vi "Load Preset.vi"(8 "error in (no error)":errorcluster, 10 "Preset Name":string, 11 "Config":T3) -> (0 "error out":errorcluster, 1 "Dump Stat":T1, 2 "Levels Available":i32, 3 "Levels":T2, 5 "No Oxy?":bool)   [LabVIEW 2021]
uses:
  <vilib>/Utility/config.llb/Config Data RefNum.ctl
  CTLs/Dump Stat.ctl
  <vilib>/Utility/config.llb/Read Key (I32).vi
  <vilib>/Utility/config.llb/NI_LVConfig.lvlib
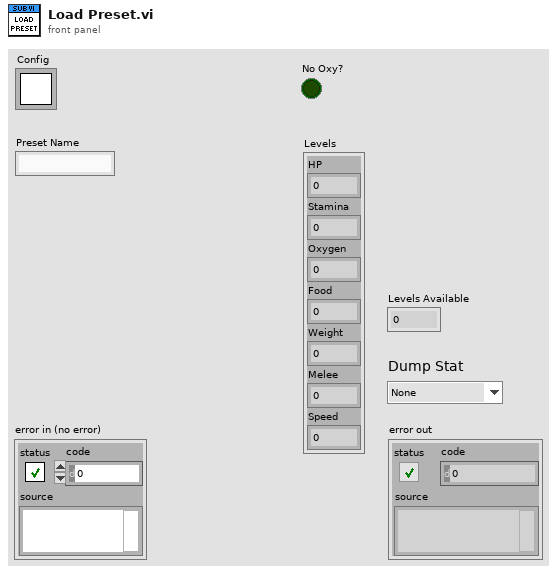
[diagram p1: front panel]
types:
  T1 = typedef "Dump Stat.ctl" = enum16{"None", "HP", "Stamina", "Oxygen", "Food", "Weight", "Melee", "Speed"}
  T2 = cluster{"HP":i32, "Stamina":i32, "Oxygen":i32, "Food":i32, "Weight":i32, "Melee":i32, "Speed":i32}
  T3 = typedef "NI_LVConfig.lvlib/Config Data RefNum.ctl" = refnum<k1>
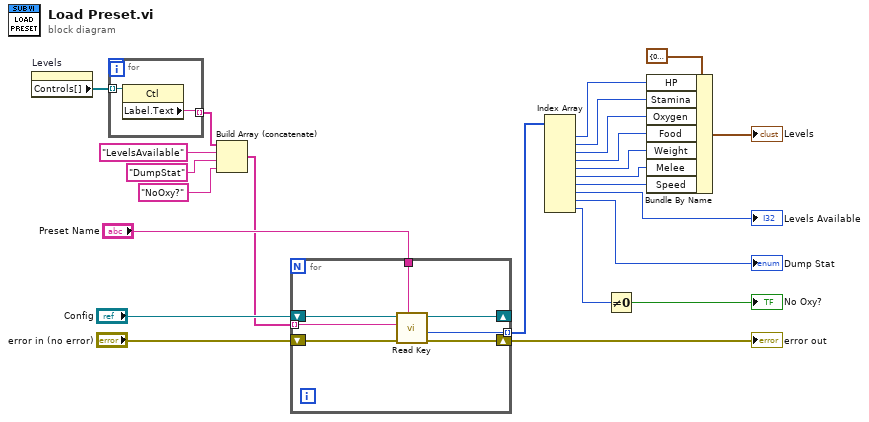
[diagram p0: block diagram]
diagram:
  n1 = property on="Levels" class="Clust (strict)"() -> ("Controls[]"=w21:refnum<vi>[])  [unwired: 2 in, 2 out]
  n2 = for {
    tunnel: w21 -> [w26] mode=indexing
    tunnel: [w25] -> w19 mode=indexing
    n3 = property class="Ctl"(reference=w26) -> ("Label.Text"=w25:string)  [unwired: 1 in, 2 out]
  }
  n4 = Build Array (concatenate)(w19, "LevelsAvailable", "DumpStat", "NoOxy?") -> (w16:string[])
  n5 = for {
    tunnel: "Preset Name" -> [w31]
    tunnel: w16 -> [w30] mode=indexing
    tunnel: [w29] -> w13 mode=indexing
    shift-right: [w28] -> w14
    shift-left: "error in (no error)" -> [w32]
    shift-right: [w27] -> _
    shift-left: "Config" -> [w33]
    n6 = call-poly <vilib>:"Read Key.vi"("section"=w31, "error in (no error)"=w32, "key"=w30, "refnum"=w33) -> ("error out"=w28:errorcluster, "value"=w29:i32, "refnum out"=w27:T3)  [unwired: 4 in, 1 out]
  }
  "error out" <- w14
  n7 = Index Array(array=w13) -> (element #1=w12:i32, element #2=w11:i32, element #3=w10:i32, element #4=w9:i32, element #5=w8:i32, element #6=w7:i32, element #7=w6:i32, element #8=→"Levels Available":i32, element #9=→"Dump Stat":i32, element #10=w5:i32)  [unwired: 10 in]
  n8 = Not Equal To 0?(x=w5) -> (x != 0?=→"No Oxy?":bool)
  n9 = Bundle By Name(cluster=T2 {"HP"=0, "Stamina"=0, "Oxygen"=0, "Food"=0, "Weight"=0, "Melee"=0, "Speed"=0} ("Levels"), "HP"=w12, "Stamina"=w11, "Oxygen"=w10, "Food"=w9, "Weight"=w8, "Melee"=w7, "Speed"=w6) -> (→"Levels":T2)
